vi "dznrm2 - Vector 2-Norm (CDB).vi"(7 "xInc":i32=1, 11 "x":cdb[](array[numeric])) -> (0 "error":i32, 3 "dznrm2":dbl)   [LabVIEW 2020, in "NI_AALBLAS.lvlib"]
doc: "Calculates the Euclidean norm of a vector."
uses:
  <vilib>/Analysis/NI_AALBLAS.lvlib
  <vilib>/Analysis/BLAS.llb/Fucntion.ctl
  <vilib>/Analysis/BLAS.llb/BLAS1 Utility(CDB).vi
panel:
  # "dznrm2=||x||"
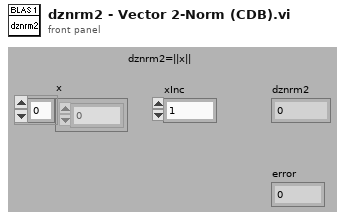
[diagram p1: front panel]
types:
  T1 = typedef "NI_AALBLAS.lvlib/Fucntion.ctl" = u16
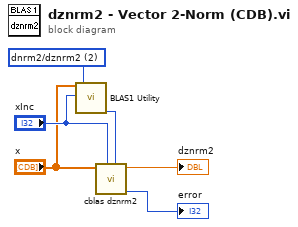
[diagram p0: block diagram]
diagram:
  w2 = T1 2 items=["ddot/zdotu/zdotc", "daxpy/zaxpy", "dnrm2/dznrm2", "dasum/dzasum", "dcopy/zcopy", "dswap/zswap", "drotm", "drot/zdrot", "idamax/izamax", "idamin/izamin", "dgemv/zgemv", "dsymv/zhemv", "dtrmv/ztrmv", "dsyr/zher", "dsyr2/zher2", "dger/zgeru/zgerc", "dtrsv/ztrsv", "dgemm/zgemm", "dsymm/zsymm/zhemm", "dtrmm/ztrmm", "dsyrk/zsyrk/zherk", "dsyr2k/zsyr2k/zher2k", "dtrsm/ztrsm"] ("function")
  n1 = call-poly <vilib>:"BLAS1 Utility.vi"("x"="x", "xInc"="xInc", "function"=w2) -> ("n"=w1:i32)  [unwired: 2 in, 14 out]
  n2 = call <vilib>:"cblas dznrm2.vi"("n"=w1, "incx"="xInc", "x"="x") -> ("error"=→"error":i32, "dznrm2"=→"dznrm2":dbl)  [unwired: 7 out]
